vi "Battery_Destroy.vi"(0 "reference in":refnum<class "Battery.lvclass">, 5 "Error In":errorcluster) -> (14 "reference out":refnum<class "Battery.lvclass">, 19 "Error Out":errorcluster)   [LabVIEW 2023, in "Battery.lvclass"]
uses:
  Battery.lvclass
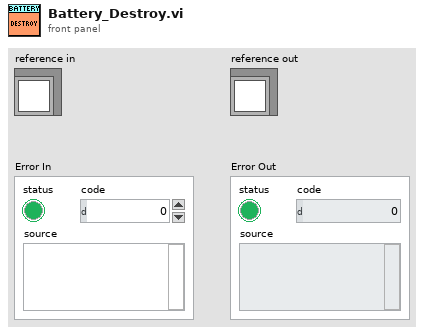
[diagram p1: front panel]
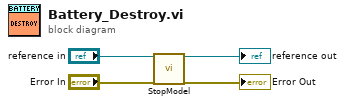
[diagram p0: block diagram]
diagram:
  n1 = call "StopModel.vi"("reference in"="reference in", "Error In"="Error In") -> ("reference out"=→"reference out":refnum<class "Battery.lvclass">, "Error Out"=→"Error Out":errorcluster)  [unwired: 16 in]
